vi "Phasor Compute tau_m SDV.vi"(6 "# Samples (1E4)":i32=10000, 8 "Error In":errorcluster, 9 "Phasor Frequency":dbl[unit], 10 "Phasor SDV (g, s)":T1, 11 "Phasor (g, s)":T1) -> (0 "Error Out":errorcluster, 1 "tau_m SDV":dbl[unit], 3 "<tau_m>":dbl[unit])   [LabVIEW 2021, in "Phasor.lvlib"]
uses:
  Phasor.lvlib
  Phasor (g, s).ctl
  <vilib>/gmath/statdist.llb/Normal Random.vi
  <vilib>/gmath/NI_Gmath.lvlib
  Error/Error.lvlib
  <vilib>/Analysis/NI_AALBase.lvlib
  Time/Time.lvlib
panel:
  out "CPU (s)":dbl
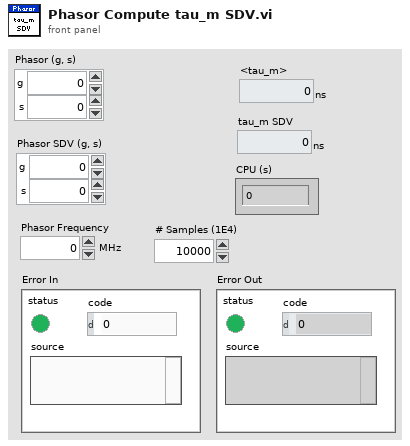
[diagram p1: front panel]
types:
  T1 = typedef "Phasor.lvlib/Phasor (g, s).ctl" = cluster{"g":dbl, "s":dbl}
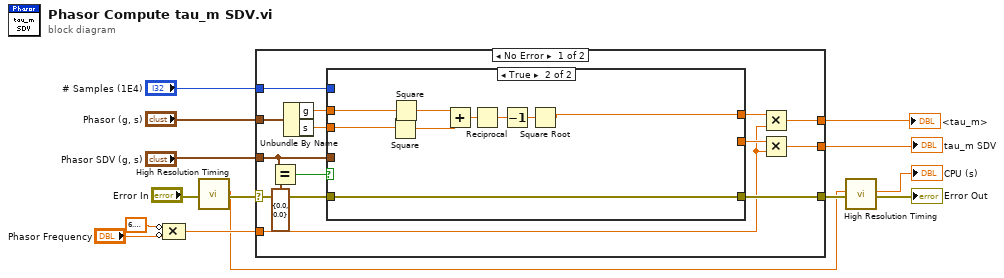
[diagram p0: block diagram]
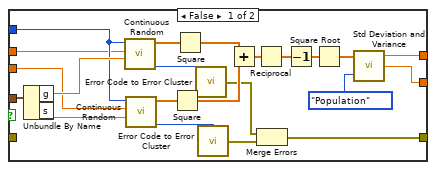
[diagram p2: hidden frame]
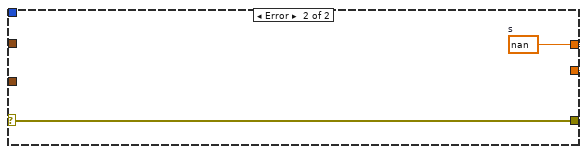
[diagram p3: hidden frame]
diagram:
  n1 = Compound Arithmetic op=MULTIPLY(invert 6.283185307179586, invert "Phasor Frequency") -> (w7:dbl[unit])
  n2 = call "High Resolution Timing.vi"("Error In"="Error In") -> ("elapsed (relative) seconds"=w2:dbl, "Error Out"=w4:errorcluster)  [unwired: 16 in, 1 out]
  n3 = case shown="No Error" w4 {
    selector: w4 -> [w15 w61]
    tunnel: "Phasor (g, s)" -> [w18 _]
    tunnel: "Phasor SDV (g, s)" -> [w21 _]
    tunnel: "# Samples (1E4)" -> [w28 _]
    tunnel: [w27 w61] -> w8
    tunnel: w7 -> [w24 _]
    tunnel: [w23 w60] -> w6
    tunnel: [w22 w60] -> w5
    frame No Error {
      n4 = Equal?(x=w21, y=T1 {"g"=0.0, "s"=0.0} ("input cluster")) -> (x = y?=w19:bool)
      n5 = Unbundle By Name(w18) -> ("g"=w17:dbl, "s"=w16:dbl)
      n6 = case shown="True" w19 {
        tunnel: w28 -> [w48 _]
        tunnel: [w34 w51] -> w27
        tunnel: [w33 w52] -> w26
        tunnel: [w32 _] -> w25
        tunnel: w21 -> [w31 _]
        tunnel: w17 -> [w30 w55]
        tunnel: w16 -> [w29 w54]
        tunnel: w15 -> [_ w51]
        frame False {
          n7 = Unbundle By Name(w31) -> ("g"=w50:dbl, "s"=w49:dbl)
          n8 = call-poly <vilib>:"Continuous Random.vi"("std"=w50, "mean"=w30, "samples"=w48) -> ("error"=w47:i32, "normal random data"=w45:dbl[])  [unwired: 7 in]
          n9 = call-poly <vilib>:"Continuous Random.vi"("std"=w49, "mean"=w29, "samples"=w48) -> ("error"=w46:i32, "normal random data"=w44:dbl[])  [unwired: 7 in]
          n10 = Square(x=w44) -> (x^2=w42:dbl[])
          n11 = Square(x=w45) -> (x^2=w43:dbl[])
          n12 = call "Error Code to Error Cluster.vi"("Error Code"=w47) -> ("Error Out"=w35:errorcluster)  [unwired: 14 in]
          n13 = call "Error Code to Error Cluster.vi"("Error Code"=w46) -> ("Error Out"=w36:errorcluster)  [unwired: 14 in]
          n14 = Add(x=w43, y=w42) -> (x+y=w41:dbl[])
          n15 = Reciprocal(x=w41) -> (1/x=w40:dbl[])
          n16 = Merge Errors(w35, w36) -> (w34:errorcluster)
          n17 = Decrement(x=w40) -> (x-1=w39:dbl[])
          n18 = Square Root(x=w39) -> (sqrt(x)=w38:dbl[])
          n19 = call <vilib>:"Std Deviation and Variance.vi"("X"=w38, "Weighting (Sample)"=enum16{"Sample", "Population"}."Population") -> ("mean"=w33:dbl, "standard deviation"=w32:dbl)  [unwired: 1 out]
        }
        frame True {
          n20 = Square(x=w54) -> (x^2=w53:dbl)
          n21 = Square(x=w55) -> (x^2=w59:dbl)
          n22 = Add(x=w59, y=w53) -> (x+y=w58:dbl)
          n23 = Reciprocal(x=w58) -> (1/x=w57:dbl)
          n24 = Decrement(x=w57) -> (x-1=w56:dbl)
          n25 = Square Root(x=w56) -> (sqrt(x)=w52:dbl)
        }
      }
      n26 = Multiply(x=w26, y=w24) -> (x*y=w22:dbl[unit])
      n27 = Multiply(x=w25, y=w24) -> (x*y=w23:dbl[unit])
    }
    frame Error {
      w60 = dbl[unit] nan  # s
    }
  }
  "tau_m SDV" <- w6
  "<tau_m>" <- w5
  n28 = call "High Resolution Timing.vi"("relative seconds (NaN)"=w2, "Error In"=w8) -> ("elapsed (relative) seconds"=→"CPU (s)":dbl, "Error Out"=→"Error Out":errorcluster)  [unwired: 15 in, 1 out]
